vi "Read T ctl driver.vi"(8 "error in (no error)":errorcluster, 11 "Temperature Controller in":refnum<class "Temperature Controller.lvclass">) -> (0 "error out":errorcluster, 2 "Temperature Controller Driver.lvclass":refnum<class "Temperature Controller Driver.lvclass">, 3 "Temperature Controller out":refnum<class "Temperature Controller.lvclass">)   [LabVIEW 2016, in "Temperature Controller.lvclass"]
uses:
  Temperature Controller.lvclass
  C:/github/LabActor/Instrument Actor/Instrument Actor.lvclass
  NHMFL_Core/Libraries/Instruments/Temperature Controller Driver/Temperature Controller Driver.lvclass
  Instrument Actor/Instrument Actor.lvclass/Instrument Actor.ctl
  Instrument Actor/Read Instrument driver.vi
  NHMFL_Core/Libraries/Instruments/Instrument Driver/Instrument Driver.lvclass
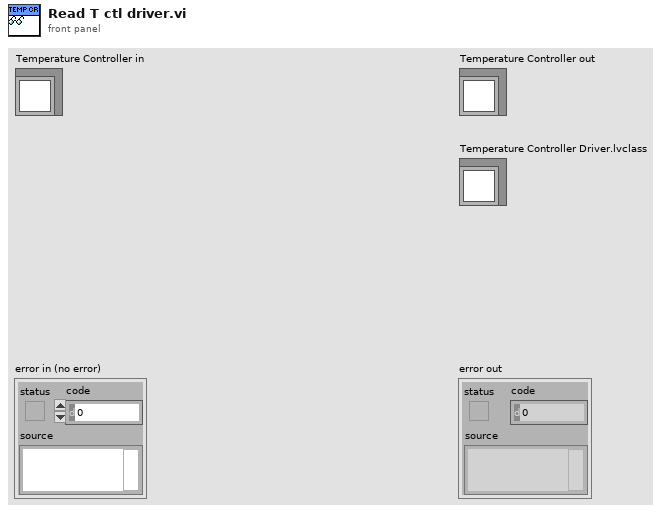
[diagram p1: front panel]
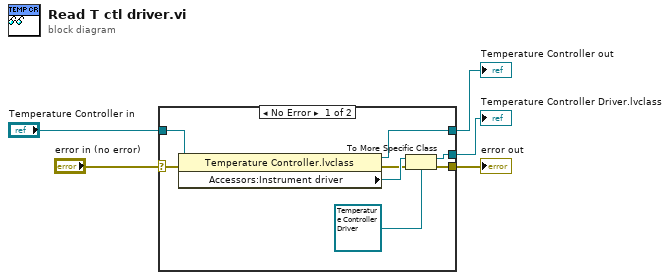
[diagram p0: block diagram]
diagram:
  n1 = case shown="No Error" "error in (no error)" {
    selector: "error in (no error)" -> [w11 w14]
    tunnel: [w7 w14] -> w4
    tunnel: [w12 w15] -> w2
    tunnel: "Temperature Controller in" -> [w13 w15]
    tunnel: [w9 _] -> w1
    frame No Error {
      n2 = property class="Temperature Controller.lvclass"(reference=w13, error in=w11) -> (reference out=w12:refnum<class "Temperature Controller.lvclass">, error out=w8:errorcluster, "Accessors:Instrument driver"=w10:refnum<class "Instrument Driver.lvclass">)
      n3 = To More Specific Class(target class=refnum<class "Temperature Controller Driver.lvclass"> refnum ("Temperature Controller Driver.lvclass"), reference=w10, error in=w8) -> (specific class reference=w9:refnum<class "Temperature Controller Driver.lvclass">, error out=w7:errorcluster)
    }
    frame Error {
    }
  }
  "error out" <- w4
  "Temperature Controller out" <- w2
  "Temperature Controller Driver.lvclass" <- w1
